vi "SubVI Function Call Parameters C Code Chunks.vi"(8 "Error In":errorcluster, 10 "VI Reference":refnum<vi>, 11 "SubVI Refnum":refnum<vi>) -> (0 "SubVI output variable name":string, 1 "SubVI func. declaration":string, 2 "return datatype":string, 3 "SubVI func. call in code":string, 4 "Error Out":errorcluster, 5 "reference out":refnum<vi>)   [LabVIEW 2014]
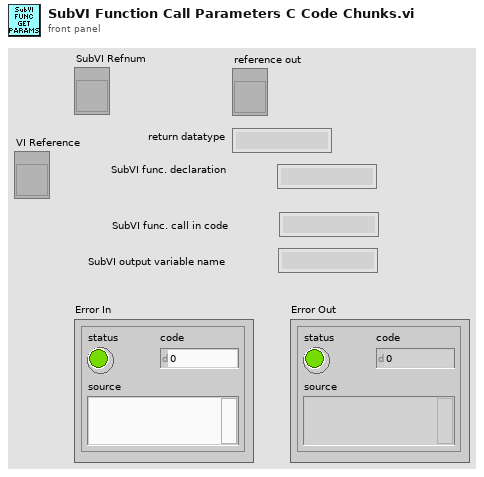
[diagram p1: front panel]
types:
  T1 = cluster{"terminals datatypes":string[][], "terminal\nconnected?":bool[], "terminal captions":string[], "term. count":i32, "terminal\nIsSource?":bool[], "SubVI name":string, "connected\nwires refs.":refnum<vi>[], "coerced dot?":bool[], "terminals[]":refnum<vi>[]}
  T2 = cluster{"wire labels":string[], "wire terminals datatypes":string[][]}
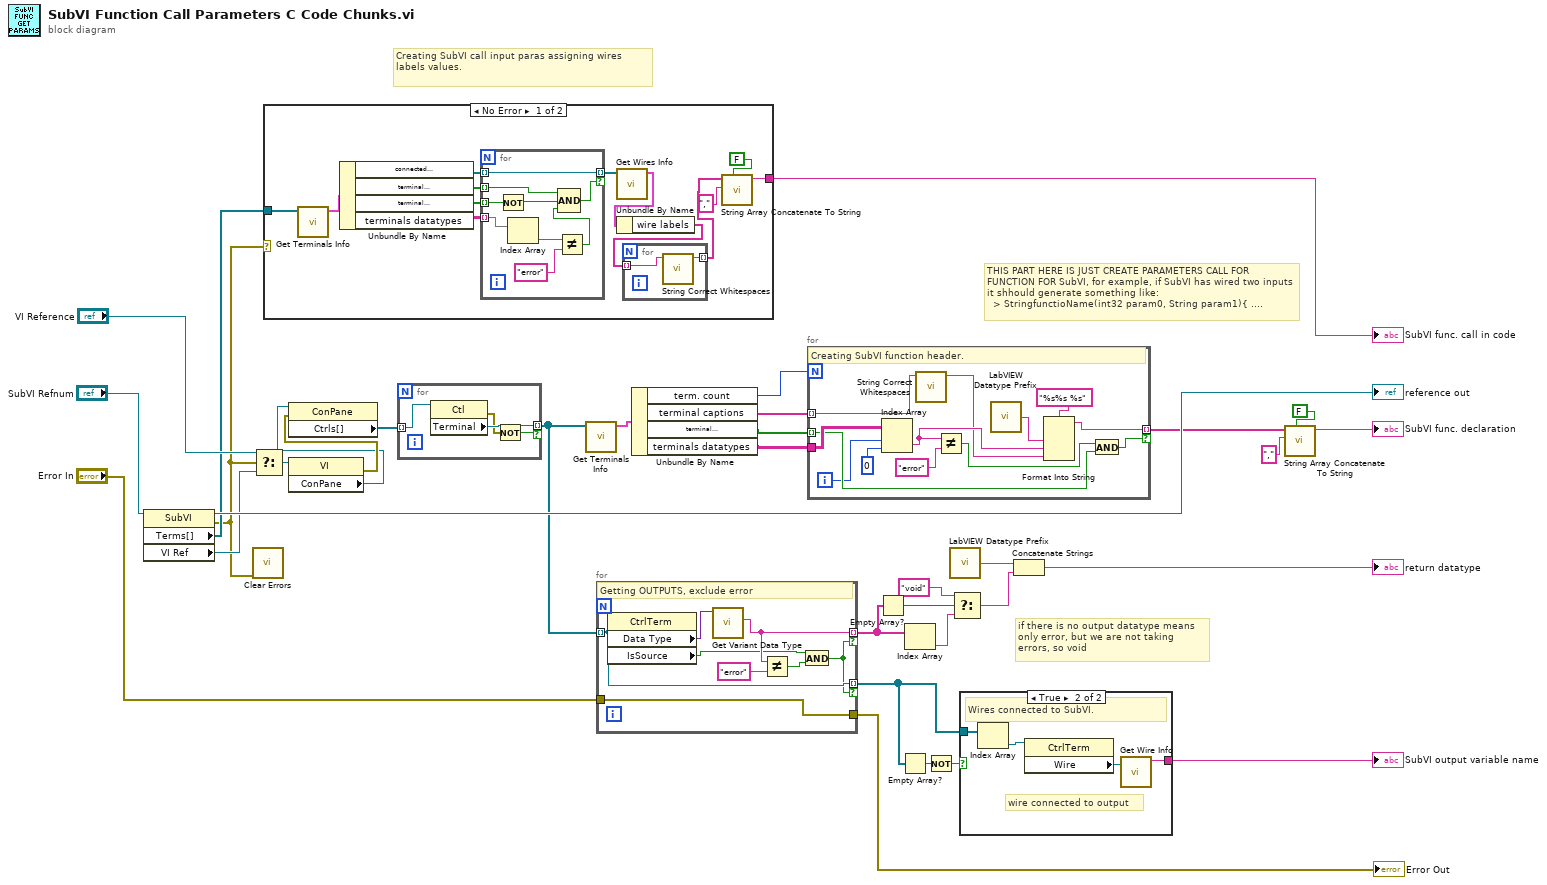
[diagram p0: block diagram]
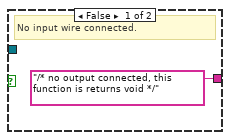
[diagram p3: hidden frame]
diagram:
  # "Creating SubVI call input paras assigning wires labels values."
  # "if there is no output datatype means only error, but we are not taking errors, so void"
  # "THIS PART HERE IS JUST CREATE PARAMETERS CALL FOR FUNCTION FOR SubVI, for example, if SubVI has wired two inputs it shhould generate something like:\n  > StringfunctioName(int32 param0, String param1){ ...."
  n1 = property class="SubVI"(reference="SubVI Refnum") -> (reference out=→"reference out":refnum<vi>, error out=w2:errorcluster, "Terms[]"=w3:refnum<vi>[], "VI Ref"=w5:refnum<vi>)  [unwired: 1 in]
  n2 = call <vilib>:"Clear Errors.vi"("error in (no error)"=w2) -> ()  [unwired: 5 in, 2 out]
  n3 = Select(t="VI Reference", s=w2, f=w5) -> (s? t:f=w4:refnum<vi>)
  n4 = case shown="No Error" w2 {
    tunnel: w3 -> [w47 _]
    tunnel: [w35 _] -> w1
    frame No Error {
      n5 = call "Get Terminals Info.vi"("Terms[]"=w47) -> ("output cluster"=w46:T1)  [unwired: 9 in, 1 out]
      n6 = Unbundle By Name(w46) -> ("connected\nwires refs."=w43:refnum<vi>[], "terminal\nconnected?"=w44:bool[], "terminal\nIsSource?"=w45:bool[], "terminals datatypes"=w42:string[][])
      n7 = for {
        tunnel: w45 -> [w58] mode=indexing
        tunnel: w44 -> [w56] mode=indexing
        tunnel: w43 -> [w55] mode=indexing
        tunnel: [w55] -> w40 mode=indexing if=w54
        tunnel: w42 -> [w52] mode=indexing
        n8 = Not(x=w58) -> (.not. x?=w57:bool)
        n9 = Index Array(array=w52) -> (element=w50:string)  [unwired: 1 in]
        n10 = Not Equal?(x=w50, y="error" ("x")) -> (x != y?=w53:bool)
        n11 = Compound Arithmetic op=AND(w56, w57, w53) -> (w54:bool)
      }
      n12 = call "Get Wires Info.vi"("connected\nwires refs."=w40) -> ("output cluster 2"=w41:T2)  [unwired: 10 in]
      n13 = Unbundle By Name(w41) -> ("wire labels"=w39:string[])
      n14 = for {
        tunnel: w39 -> [w49] mode=indexing
        tunnel: [w48] -> w36 mode=indexing
        n15 = call "String Correct Whitespaces.vi"("String in"=w49) -> ("String out"=w48:string)  [unwired: 10 in]
      }
      n16 = call "String Array Concatenate To String.vi"("insert last delimiter?"=FALSE, "Delimiter char"=",", "Array String In"=w36) -> ("String"=w35:string)  [unwired: 8 in]
    }
    frame Error {
    }
  }
  "SubVI func. call in code" <- w1
  n17 = property class="VI"(reference=w4) -> (error out=w10:errorcluster, "ConPane"=w9:refnum<vi>)  [unwired: 1 in, 1 out]
  n18 = property class="ConPane"(reference=w9, error in=w10) -> ("Ctrls[]"=w8:refnum<vi>[])  [unwired: 2 out]
  n19 = for {
    tunnel: w8 -> [w62] mode=indexing
    tunnel: [w61] -> w7 mode=indexing if=w60
    n20 = property class="Ctl"(reference=w62) -> (error out=w59:errorcluster, "Terminal"=w61:refnum<vi>)  [unwired: 1 in, 1 out]
    n21 = Not(x=w59) -> (.not. x?=w60:bool)
  }
  n22 = call "Get Terminals Info.vi"("Terms[]"=w7) -> ("output cluster"=w16:T1)  [unwired: 9 in, 1 out]
  n23 = for {
    tunnel: [w69] -> w28 mode=indexing if=w64
    tunnel: w7 -> [w65] mode=indexing
    tunnel: [w65] -> w21 mode=indexing if=w64
    tunnel: [w63] -> w18
    tunnel: "Error In" -> [w63]
    # "Getting OUTPUTS, exclude error"
    n24 = property class="CtrlTerm"(reference=w65) -> ("Data Type"=w70:variant, "IsSource"=w66:bool)  [unwired: 1 in, 2 out]
    n25 = call "Get Variant Data Type.vi"("Variant in"=w70) -> ("first data type"=w69:string)  [unwired: 9 in, 1 out]
    n26 = Not Equal?(x=w69, y="error") -> (x != y?=w67:bool)
    n27 = And(x=w66, y=w67) -> (x .and. y?=w64:bool)
  }
  "Error Out" <- w18
  n28 = Unbundle By Name(w16) -> ("term. count"=w15:i32, "terminal captions"=w14:string[], "terminal\nIsSource?"=w13:bool[], "terminals datatypes"=w12:string[][])
  n29 = for {
    N: w15 -> [_]
    tunnel: w14 -> [w74] mode=indexing
    tunnel: w13 -> [w77] mode=indexing
    tunnel: w12 -> [w82]
    tunnel: [w79] -> w11 mode=indexing if=w72
    i -> [w71]
    # "Creating SubVI function header."
    n30 = Index Array(array=w82, index (row)=w71, index (col)=0 ("disabled index (col)")) -> (element=w76:string)
    n31 = call "String Correct Whitespaces.vi"("String in"=w74) -> ("String out"=w73:string)  [unwired: 10 in]
    n32 = Not Equal?(x=w76, y="error") -> (x != y?=w78:bool)
    n33 = call "LabVIEW Datatype Prefix.vi"() -> ("datatype prefix"=w75:string)
    n34 = Format Into String(format string="%s%s %s", w75, w76, w73) -> (resulting string=w79:string)  [unwired: 2 in, 1 out]
    n35 = And(x=w78, y=w77) -> (x .and. y?=w72:bool)
  }
  n36 = Empty Array?(array=w28) -> (empty?=w29:bool)
  n37 = Empty Array?(array=w21) -> (empty?=w22:bool)
  n38 = Index Array(array=w28) -> (element=w27:string)  [unwired: 1 in]
  n39 = Not(x=w22) -> (.not. x?=w20:bool)
  n40 = call "LabVIEW Datatype Prefix.vi"() -> ("datatype prefix"=w31:string)
  n41 = Select(t="void", s=w29, f=w27) -> (s? t:f=w25:string)
  n42 = case shown="True" w20 {
    tunnel: w21 -> [_ w88]
    tunnel: ["/* no output connected, this function is returns void */" ("wire label") w85] -> w23
    frame False {
      # "No input wire connected."
    }
    frame True {
      # "wire connected to output"
      # "Wires connected to SubVI."
      n43 = Index Array(array=w88) -> (element=w87:refnum<vi>)  [unwired: 1 in]
      n44 = property class="CtrlTerm"(reference=w87) -> ("Wire"=w86:refnum<vi>)  [unwired: 1 in, 2 out]
      n45 = call "Get Wire Info.vi"("Wire"=w86) -> ("wire label"=w85:string)  [unwired: 9 in, 1 out]
    }
  }
  "SubVI output variable name" <- w23
  n46 = Concatenate Strings(w31, w25) -> (→"return datatype":string)
  n47 = call "String Array Concatenate To String.vi"("insert last delimiter?"=FALSE, "Delimiter char"=",", "Array String In"=w11) -> ("String"=→"SubVI func. declaration":string)  [unwired: 8 in]
